vi "Global.vi"() -> ()   [LabVIEW 2011]
panel:
  in  "GlobalWarnings":string
  in  "GlobalRate8":i32
  in  "GlobalRate7":i32
  in  "GlobalRate6":i32
  in  "GlobalRate5":i32
  in  "GlobalRate4":i32
  in  "GlobalRate3":i32
  in  "GlobalRate2":i32
  in  "GlobalRate1":i32
  in  "GlobalSyncRate":i32
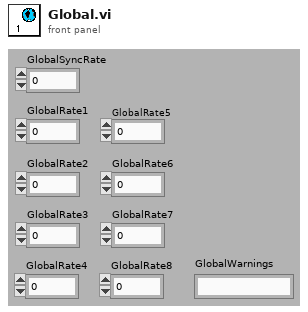
[diagram p1: front panel]
diagram:
